vi "Get Child Info.vi"(8 "error in (no error)":errorcluster, 11 "Data Value Reference in":refnum<data-value>) -> (0 "error out":errorcluster, 2 "Instance Identifier":string[](array[string]), 3 "Display Names":string[](array[string]))   [LabVIEW 2013, in "Standard Engine Editor Node.lvclass"]
uses:
  Standard Engine Editor Node.lvclass
  <vilib>/NI/Configuration Framework/Node/NISE_CEF_Node.lvclass/NISE_CEF_Node.ctl
  <vilib>/NI/Tag Bus Data Framework/Configuration Editor/Classes/Module editor node/module editor node.lvclass
  <vilib>/NI/Configuration Framework/serializable configuration/NISE_CEF_serializable configuration.lvclass/NISE_CEF_serializable configuration.ctl
  <vilib>/NI/Configuration Framework/serializable configuration/NISE_CEF_serializable configuration.lvclass
  <vilib>/NI/Configuration Framework/serializable configuration/Read UID.vi
  <vilib>/NI/Configuration Framework/Node/ReadChildren.vi
  <vilib>/NI/Tag Bus Data Framework/Configuration Editor/Classes/Module editor node/Read Module Configuration.vi
  <vilib>/NI/Configuration Framework/serializable configuration/get alias.vi
  <vilib>/NI/Configuration Framework/Node/NISE_CEF_Node.lvclass
  <vilib>/NI/Tag Bus Module Framework/module configuration/TBM module configuration.lvclass
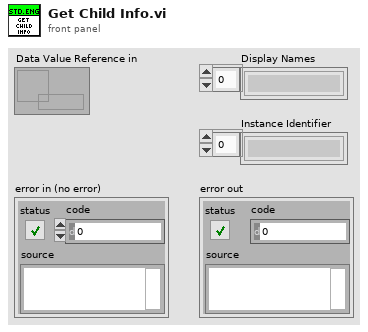
[diagram p1: front panel]
types:
  T1 = typedef "NISE_CEF_Node.lvclass/NodeRef.ctl" = refnum<data-value>
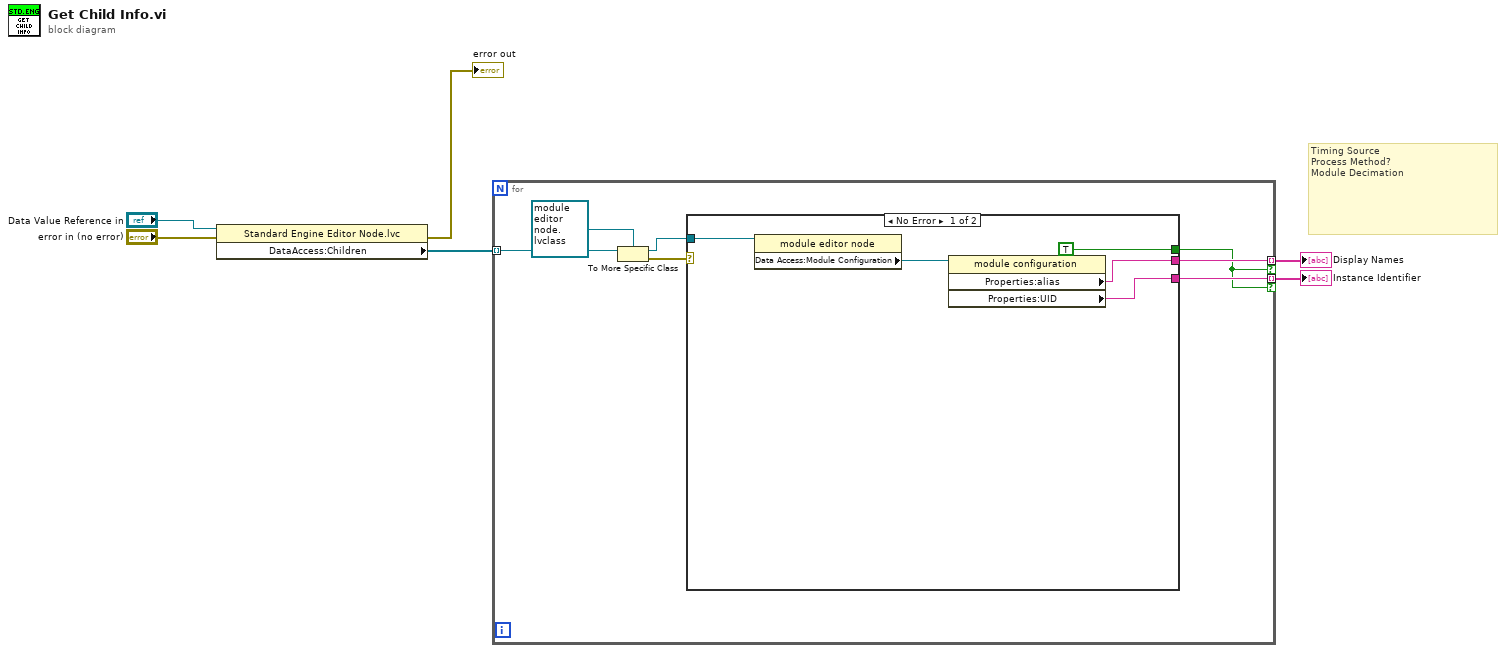
[diagram p0: block diagram]
diagram:
  # "Timing Source\nProcess Method?\nModule Decimation"
  n1 = property class="Standard Engine Editor Node.lvc"(reference="Data Value Reference in", error in="error in (no error)") -> (error out=→"error out":errorcluster, "DataAccess:Children"=w1:T1[])  [unwired: 1 out]
  n2 = for {
    tunnel: w1 -> [w13] mode=indexing
    tunnel: [w9] -> w5 mode=indexing if=w7
    tunnel: [w8] -> w6 mode=indexing if=w7
    n3 = To More Specific Class(target class=refnum<data-value> refnum ("data value reference"), reference=w13) -> (specific class reference=w10:refnum<data-value>, error out=w12:errorcluster)  [unwired: 1 in]
    n4 = case shown="No Error" w12 {
      tunnel: w10 -> [w18 _]
      tunnel: [w14 _] -> w9
      tunnel: [TRUE _] -> w7
      tunnel: [w15 _] -> w8
      frame No Error {
        n5 = property class="module editor node"(reference=w18) -> ("Data Access:Module Configuration"=w16:refnum<class "TBM module configuration.lvclass">)  [unwired: 1 in, 2 out]
        n6 = property class="module configuration"(reference=w16) -> ("Properties:alias"=w14:string, "Properties:UID"=w15:string)  [unwired: 1 in, 2 out]
      }
      frame Error {
      }
    }
  }
  "Instance Identifier" <- w6
  "Display Names" <- w5
